vi "PageChanging.vi"(1 "Pages":bool[](array[boolean])) -> (0 "Tab Control":enum32{"Page 1", "Page 2"}(tab))   [LabVIEW 2018]
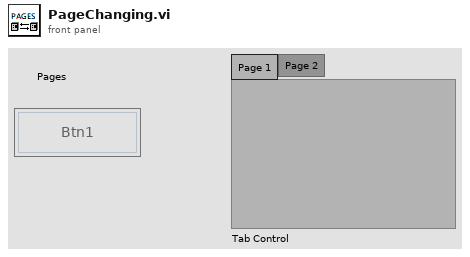
[diagram p1: front panel]
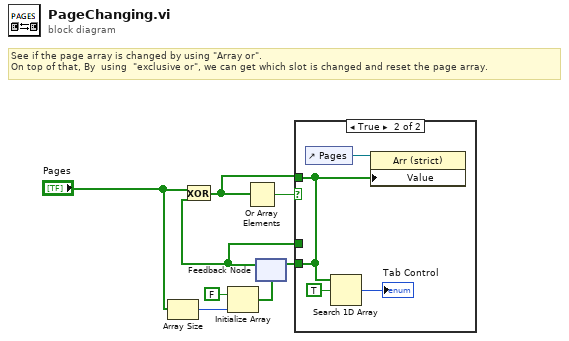
[diagram p0: block diagram]
diagram:
  # "See if the page array is changed by using \"Array or\".\nOn top of that, By  using  \"exclusive or\", we can get which slot is changed and reset the page array."
  n1 = Array Size(array="Pages") -> (size(s)=w6:i32)
  n2 = Initialize Array(FALSE, w6) -> (w5:bool[])
  n3 = feedback #1(w5) -> (w2:bool[])
  n4 = Exclusive Or(1:w2, 2:"Pages") -> (0:w3:bool[])
  n5 = Or Array Elements(Boolean array=w3) -> (logical OR=w4:bool)
  n6 = case shown="True" w4 {
    tunnel: [w9 w11] -> w8
    tunnel: w2 -> [w9 _]
    tunnel: w3 -> [_ w11]
    frame False {
    }
    frame True {
      n7 = control-ref of="Pages"() -> (w12:refnum<vi>)
      n8 = Search 1D Array(1D array=w11, element=TRUE) -> (index of element=→"Tab Control":i32)  [unwired: 1 in]
      n9 = property class="Arr (strict)"(reference=w12, "Value"=w11) -> ()  [unwired: 1 in, 2 out]
    }
  }
  n10 = feedback-in #1(w8) -> ()
